vi "Analysis.vi"(0 "Voltage":dbl[](array[numeric]) format="%.2f", 5 "Current":dbl[](array[numeric]) format="%.2f", 11 "error in (no error)":errorcluster, 13 "Create Analysis?":bool) -> (4 "Analyzed Data":T1, 15 "error out":errorcluster)   [LabVIEW 2021, in "Power Measurement_Z Power Module.lvlib"]
uses:
  Power Measurement_Z Power Module.lvlib
  Typedefs/Pow Meas Analyzed Data.ctl
  Main Library_Z Power Module.lvlib
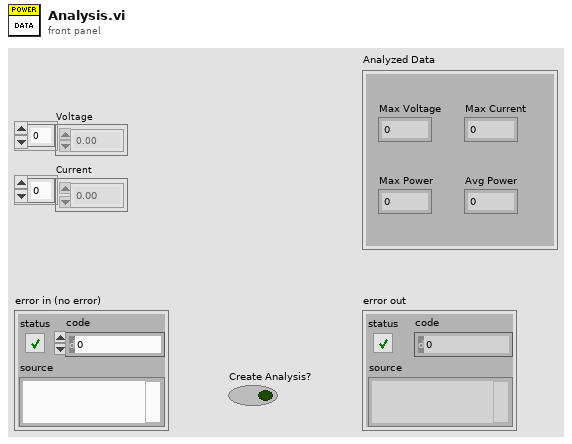
[diagram p1: front panel]
types:
  T1 = typedef "Main Library_Z Power Module.lvlib/Pow Meas Analyzed Data.ctl" = cluster{"Max Voltage":dbl, "Max Current":dbl, "Max Power":dbl, "Avg Power":dbl}
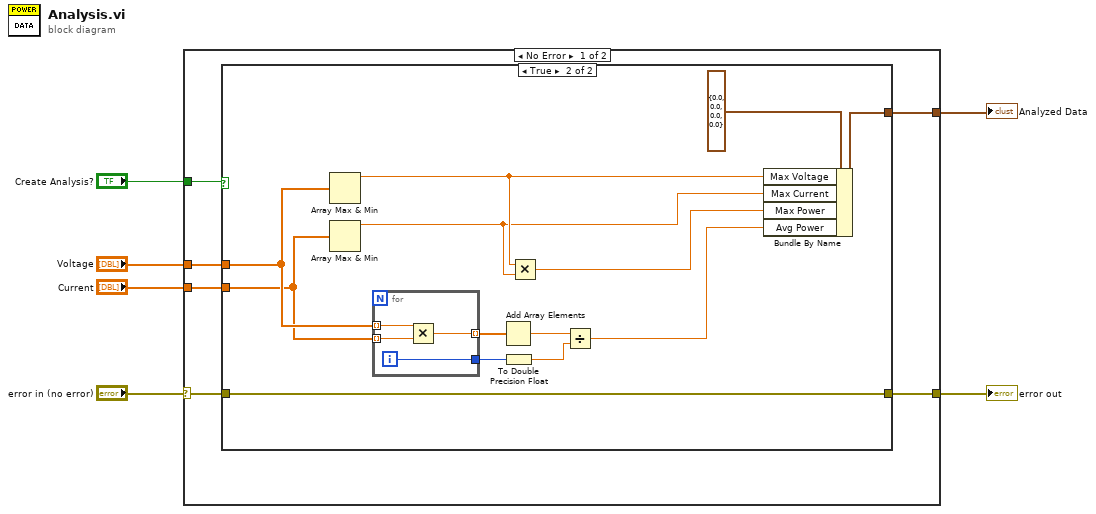
[diagram p0: block diagram]
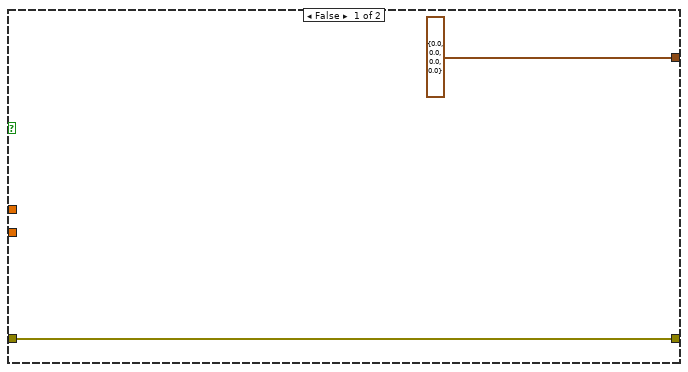
[diagram p2: hidden frame]
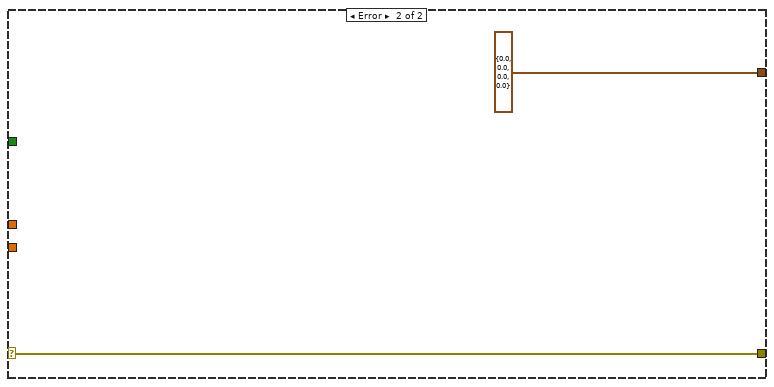
[diagram p3: hidden frame]
diagram:
  n1 = case shown="No Error" "error in (no error)" {
    selector: "error in (no error)" -> [w9 w32]
    tunnel: "Voltage" -> [w12 _]
    tunnel: "Current" -> [w11 _]
    tunnel: [w10 T1 {"Max Voltage"=0.0, "Max Current"=0.0, "Max Power"=0.0, "Avg Power"=0.0} ("Analyzed Data")] -> w4
    tunnel: [w8 w32] -> w3
    tunnel: "Create Analysis?" -> [w7 _]
    frame No Error {
      n2 = case shown="True" w7 {
        tunnel: w12 -> [_ w27]
        tunnel: w11 -> [_ w26]
        tunnel: [T1 {"Max Voltage"=0.0, "Max Current"=0.0, "Max Power"=0.0, "Avg Power"=0.0} ("Analyzed Data") w24] -> w10
        tunnel: w9 -> [w13 w15]
        tunnel: [w13 w15] -> w8
        frame False {
        }
        frame True {
          n3 = Array Max & Min(array=w27) -> (max value=w23:dbl)  [unwired: 3 out]
          n4 = Array Max & Min(array=w26) -> (max value=w22:dbl)  [unwired: 3 out]
          n5 = for {
            tunnel: w27 -> [w31] mode=indexing
            tunnel: w26 -> [w30] mode=indexing
            tunnel: [w29] -> w19 mode=indexing
            tunnel: [w28] -> w17
            i -> [w28]
            n6 = Multiply(x=w31, y=w30) -> (x*y=w29:dbl)
          }
          n7 = Add Array Elements(numeric array=w19) -> (sum=w18:dbl)
          n8 = To Double Precision Float(number=w17) -> (double precision float=w16:dbl)
          n9 = Multiply(x=w23, y=w22) -> (x*y=w21:dbl)
          n10 = Divide(x=w18, y=w16) -> (x/y=w20:dbl)
          n11 = Bundle By Name(cluster=T1 {"Max Voltage"=0.0, "Max Current"=0.0, "Max Power"=0.0, "Avg Power"=0.0} ("Analyzed Data"), "Max Voltage"=w23, "Max Current"=w22, "Max Power"=w21, "Avg Power"=w20) -> (w24:T1)
        }
      }
    }
    frame Error {
    }
  }
  "error out" <- w3
  "Analyzed Data" <- w4
